vi "Spindexer_Globals.vi"() -> ()   [LabVIEW 2019]
uses:
  Subsystems/Spindexer/Spindexer_modes.ctl
  Subsystems/Spindexer/Spindexer_Cluster.ctl
panel:
  in  "Spindexer_Set_Notifier":refnum<notifier>
  in  "Spindexer_Execute_Notifier":refnum<notifier>
  in  "Spindexer_Execute_Ref":string
  in  "Spindexer_Set_Ref":string
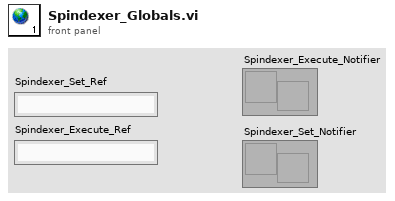
[diagram p1: front panel]
diagram:
